vi "Target Prosthesis Control System.vi"() -> (3 "Target Sensors":T1, 4 "Stop":bool)   [LabVIEW 2018]
uses:
  Ankle Benchtop Testing Advanced/Target Sensors.ctl
  Ankle Benchtop Testing Advanced/Target Raw Sensors.ctl
  Ankle Benchtop Testing Advanced/Target Filtered Sensors.ctl
  Kollmorgen Motor Control/COBRA Kollmorgen Motor IO Library.lvlib
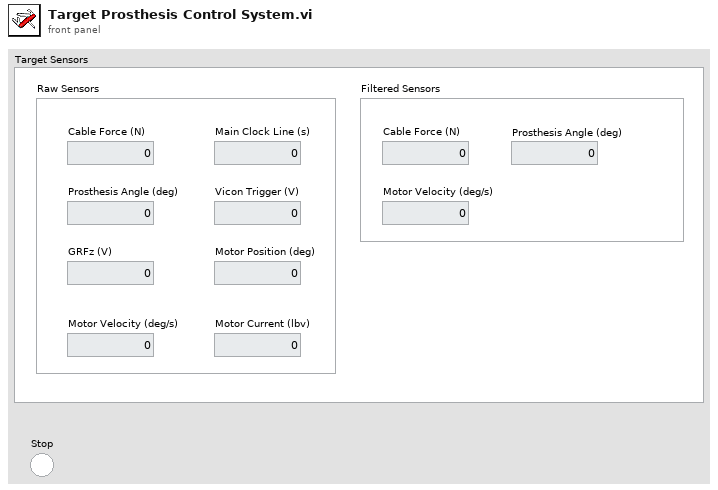
[diagram p1: front panel]
types:
  T1 = typedef "Target Sensors.ctl" = cluster{"Raw Sensors":T2, "Filtered Sensors":T3}
  T2 = typedef "Target Raw Sensors.ctl" = cluster{"Cable Force (N)":dbl, "Prosthesis Angle (deg)":dbl, "Main Clock Line (s)":dbl, "Vicon Trigger (V)":dbl, "GRFz (V)":dbl, "Motor Position (deg)":dbl, "Motor Velocity (deg/s)":dbl, "Motor Current (lbv)":dbl}
  T3 = typedef "Target Filtered Sensors.ctl" = cluster{"Cable Force (N)":dbl, "Prosthesis Angle (deg)":dbl, "Motor Velocity (deg/s)":dbl}
  T4 = typedef "Target Gait Phase Data.ctl" = cluster{"Phase":dbl, "HS":bool, "Filtered GRFz (N)":dbl, "GRFz Rate (N/s)":dbl}
  T5 = typedef "Target Cable Force Setpoint Data.ctl" = cluster{"Cable Force Setpoint (N)":dbl, "Spring Torque (Nm)":dbl, "Prosthesis Lever Arm (m)":dbl}
  T6 = cluster{"Motor Velocity Command (deg/s)":dbl, "Feedback Contribution (deg/s)":dbl, "ILC Contribution (deg/s)":dbl}
  T7 = typedef "COBRA Kollmorgen Motor IO Library.lvlib/Target Motor Command Options.ctl" = enum16{"Current Command", "Velocity Command"}
  T8 = cluster{"Command Type":T7, "Motor Velocity Command (deg/s)":dbl}
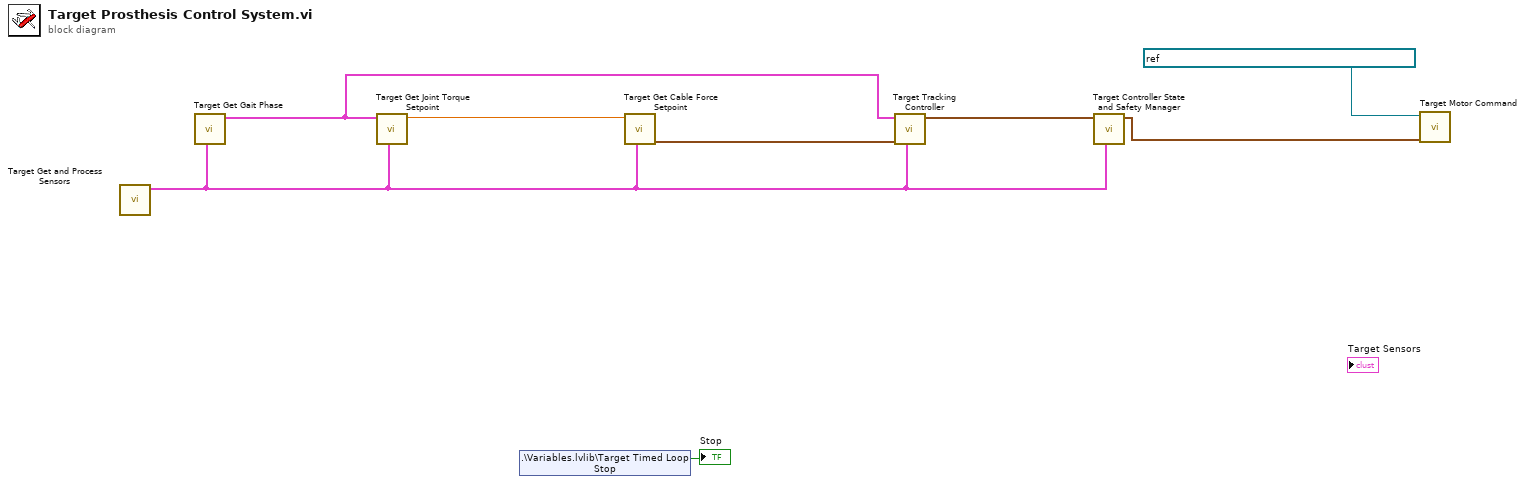
[diagram p0: block diagram]
diagram:
  n1 = call "Target Get and Process Sensors.vi"() -> ("Target Sensors"=w3:T1)  [unwired: 11 in]
  n2 = call "Target Get Gait Phase.vi"("Target Sensors"=w3) -> ("Gait Phase Data"=w6:T4)  [unwired: 10 in]
  n3 = call "Target Get Joint Torque Setpoint.vi"("Target Sensors"=w3, "Gait Phase Data"=w6) -> ("Joint Torque Setpoint (Nm)"=w7:dbl)  [unwired: 9 in]
  n4 = shared-variable ".\\Variables.lvlib\\Target Timed Loop Stop"() -> (→"Stop":bool)  [unwired: 1 in, 1 out]
  n5 = call "Target Get Cable Force Setpoint.vi"("Target Sensors"=w3, "Joint Torque Setpoint (Nm)"=w7) -> ("Cable Force Setpoint Data"=w5:T5)  [unwired: 9 in]
  n6 = call "Target Tracking Controller.vi"("Target Sensors"=w3, "Cable Force Setpoint Data"=w5, "Gait Phase Data"=w6) -> ("Controller Ouputs"=w4:T6)  [unwired: 8 in]
  n7 = call "Target Controller State and Safety Manager.vi"("Target Sensors"=w3, "Controller Ouputs"=w4) -> ("Motor Instructions"=w2:T8)  [unwired: 9 in]
  n8 = call "Target Motor Command.vi"("Motor Instructions"=w2, "Motion Handle"=refnum<k21> "nism://NI-PXIe8880-2F1836AB/AKM74L Motor") -> ()  [unwired: 10 in]
